vi "Add Extra position.vi"(4 "Positions":dbl[][](array[numeric])) -> (0 "Additional Point":dbl[](array[numeric]))   [LabVIEW 2022 SP3]
panel:
  out "Waveform Graph":dbl[][](graph)
  out "XY Graph":T1(graph)
  out "max value":dbl
  out "sorted array":dbl[][](array[numeric]) format="%.2f"
  out "changes":dbl[](array[numeric])
  # "X              Y                    Z                         C"
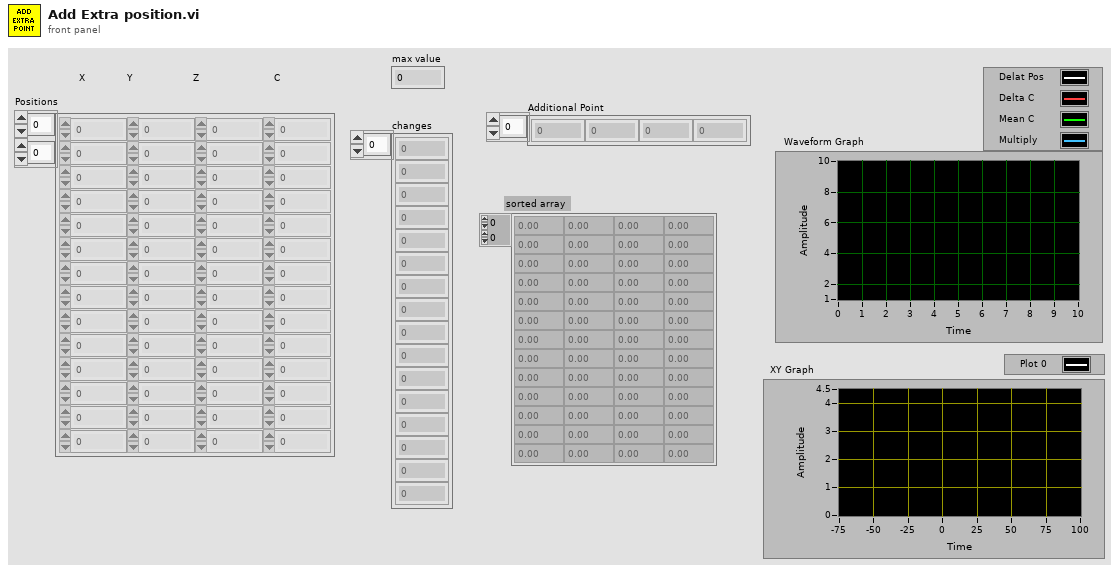
[diagram p1: front panel]
types:
  T1 = cluster{"sorted array":dbl[], "sorted array":dbl[]}
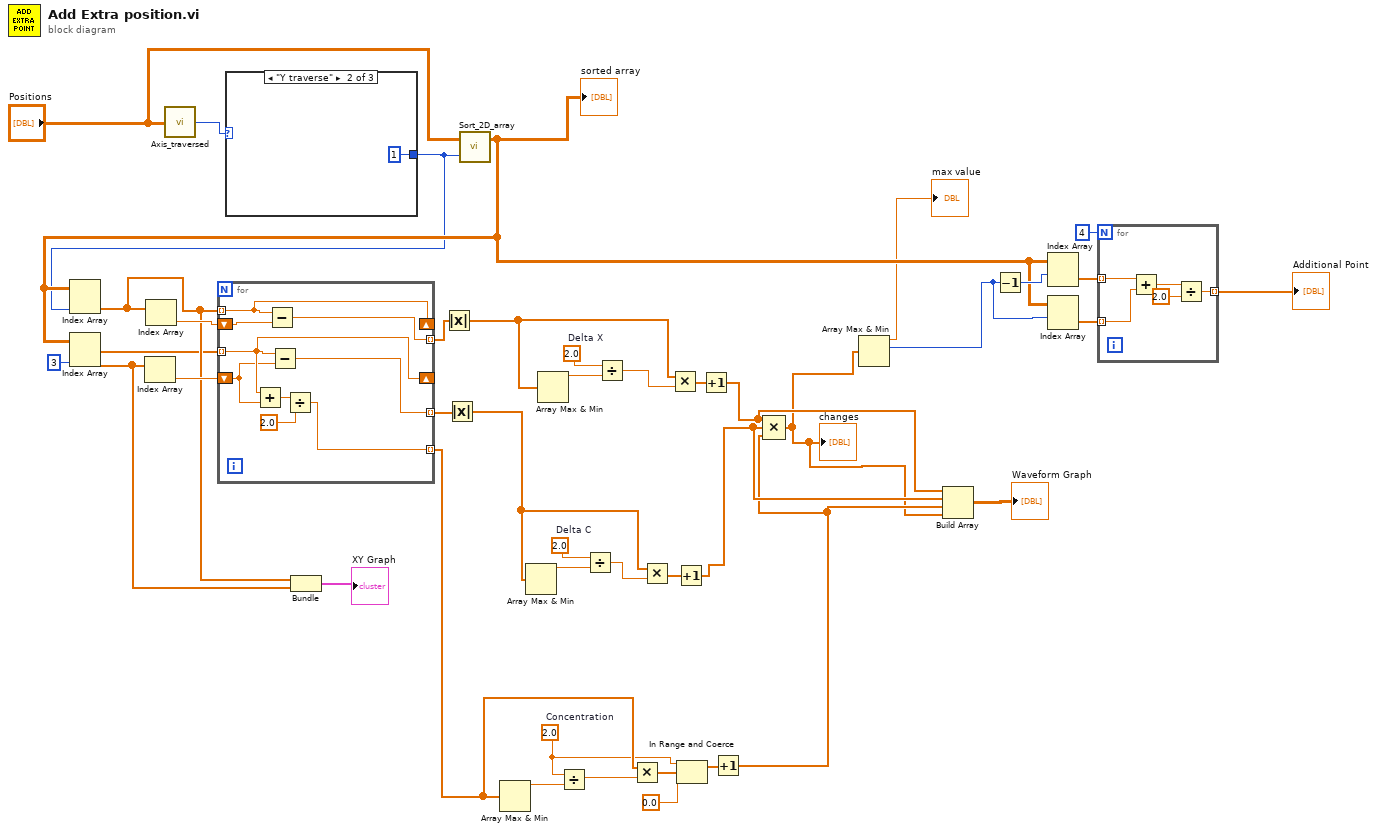
[diagram p0: block diagram]
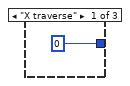
[diagram p2: hidden frame]
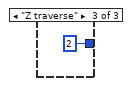
[diagram p3: hidden frame]
diagram:
  w10 = 2.0  # Delta X
  w9 = 2.0  # Delta C
  w11 = 2.0  # Concentration
  n1 = call "Axis_traversed.vi"("Position array"="Positions") -> ("Axis Traversed"=w40:enum16{"X traverse", "Y traverse", "Z traverse"})  [unwired: 4 out]
  n2 = case shown="\"Y traverse\"" w40 {
    tunnel: [0 ("disabled index (col)") 1 ("disabled index (col)") 2 ("disabled index (col)")] -> w30
    frame "X traverse" {
    }
    frame "Y traverse" {
    }
    frame "Z traverse" {
    }
  }
  n3 = call "Sort_2D_array.vi"("Column index to sort on"=w30, "unsorted array"="Positions") -> ("sorted array"=w31:dbl[][])  [unwired: 1 out]
  "sorted array" <- w31
  n4 = Index Array(array=w31, index (col)=w30) -> (element=w8:dbl[])  [unwired: 1 in]
  n5 = Index Array(array=w31, index (col)=3 ("disabled index (col)")) -> (element=w7:dbl[])  [unwired: 1 in]
  n6 = Index Array(array=w7) -> (element=w41:dbl)  [unwired: 1 in]
  n7 = Index Array(array=w8) -> (element=w29:dbl)  [unwired: 1 in]
  n8 = for {
    shift-right: [w50] -> _
    shift-left: w41 -> [w49]
    tunnel: w7 -> [w50] mode=indexing
    tunnel: [w53] -> w28 mode=indexing
    shift-right: [w52] -> _
    shift-left: w29 -> [w51]
    tunnel: w8 -> [w52] mode=indexing
    tunnel: [w46] -> w25 mode=indexing
    tunnel: [w45] -> w16 mode=indexing
    n9 = Add(x=w50, y=w49) -> (x+y=w48:dbl)
    n10 = Subtract(x=w52, y=w51) -> (x-y=w45:dbl)
    n11 = Subtract(x=w50, y=w49) -> (x-y=w53:dbl)
    n12 = Divide(x=w48, y=2.0) -> (x/y=w46:dbl)
  }
  n13 = Bundle("sorted array"=w8, "sorted array"=w7) -> (→"XY Graph":T1)  [unwired: 1 in]
  n14 = Absolute Value(x=w16) -> (abs(x)=w19:dbl[])
  n15 = Absolute Value(x=w28) -> (abs(x)=w20:dbl[])
  n16 = Array Max & Min(array=w25) -> (max value=w27:dbl)  [unwired: 3 out]
  n17 = Array Max & Min(array=w20) -> (max value=w21:dbl)  [unwired: 3 out]
  n18 = Array Max & Min(array=w19) -> (max value=w18:dbl)  [unwired: 3 out]
  n19 = Divide(x=w11, y=w27) -> (x/y=w26:dbl)
  n20 = Divide(x=w9, y=w21) -> (x/y=w22:dbl)
  n21 = Divide(x=w10, y=w18) -> (x/y=w17:dbl)
  n22 = Multiply(x=w25, y=w26) -> (x*y=w24:dbl[])
  n23 = Multiply(x=w20, y=w22) -> (x*y=w13:dbl[])
  n24 = Multiply(x=w19, y=w17) -> (x*y=w14:dbl[])
  n25 = Increment(x=w13) -> (x+1=w3:dbl[])
  n26 = In Range and Coerce(upper limit=w11, x=w24, lower limit=0.0) -> (coerced(x)=w12:dbl[])  [unwired: 1 out]
  n27 = Increment(x=w14) -> (x+1=w4:dbl[])
  n28 = Increment(x=w12) -> (x+1=w2:dbl[])
  n29 = Compound Arithmetic op=MULTIPLY(w4, w3, w2) -> (w1:dbl[])
  "changes" <- w1
  n30 = Array Max & Min(array=w1) -> (max value=→"max value":dbl, max index (indices)=w34:i32)  [unwired: 2 out]
  n31 = Build Array(w4, w3, w2, w1) -> (→"Waveform Graph":dbl[][])
  n32 = Decrement(x=w34) -> (x-1=w33:i32)
  n33 = Index Array(array=w31, index (row)=w33) -> (element=w36:dbl[])  [unwired: 1 in]
  n34 = Index Array(array=w31, index (row)=w34) -> (element=w35:dbl[])  [unwired: 1 in]
  n35 = for {
    N: 4 -> [_]
    tunnel: w36 -> [w58] mode=indexing
    tunnel: w35 -> [w57] mode=indexing
    tunnel: [w54] -> w37 mode=indexing
    n36 = Add(x=w58, y=w57) -> (x+y=w56:dbl)
    n37 = Divide(x=w56, y=2.0) -> (x/y=w54:dbl)
  }
  "Additional Point" <- w37
